vi "Energy Feedback Information Systems.vi"() -> ()   [LabVIEW 2014]
panel:
  in  "Path to Image":path=path "P:/My Documents/Demola/Naveen/Capture.PNG"
  out "t(s)":dbl
  in  "from 0s":bool
  in  "?":T1(tab)
  out "Suggested Actions":string
  out "Oil temperature meter":dbl(knob) scale=0.0..100.0
  out "Fuel meter":dbl(knob) scale=0.0..100.0
  out "Fuel Rate":dbl(slide) scale=0.0..75.0
  out "Bucket Fill (%)":dbl(knob) scale=0.0..100.0
  out "RPM Gauge":dbl(knob) scale=0.0..3000.0
  in  "Choose Excavator":string(combo)
  in  "Choose Cycles":u16(ring) items=["32", "16", "8", "4", "2", "1", ""]
  in  "Choose Driver":string(combo)
  out "Fuel Efficiency, [Kg/l]":cluster{dbl[], dbl[]}(graph)
  out "Torque/RPM Graph":cluster{dbl[], dbl[]}(graph)
  out "Time Productivity, [Kg/s]":cluster{dbl[], dbl[]}(graph)
  out "Dependence of best fuel consumption on engine RPM":i32[](graph)
  out "Dependencies of fuel consumption on filling % for 0 rpm Graph":i32[](graph)
  out "Dependence of best time productivity on engine RPM":i32[](graph)
  out "Dependencies of time productivity on filling % for 0 rpm":i32[](graph)
  out "Best Engine RPM":string
  out "Best filling %":string
  in  "Blank Button 2":bool
  in  "Blank Button":bool
  in  "Save Button 5":bool
  in  "Save Button 4":bool
  in  "Save Button 3":bool
  in  "Save Button 2":bool
  in  "Save Button":bool
  in  "String 6":string
  in  "String 5":string
  in  "String 4":string
  in  "String 3":string
  in  "Combo Box 5":string(combo)
  in  "Combo Box 4":string(combo)
  in  "Combo Box 3":string(combo)
  in  "Combo Box 2":string(combo)
  in  "Combo Box":string(combo)
  in  "String 2":string
  out "Check 1":dbl format="%#_10g"
  out "Check 4":dbl format="%#_10g"
  out "Check 2":dbl format="%#_10g"
  out "step":dbl
  out "Check 3":dbl format="%#_10g"
  out "millisecond timer value":u32
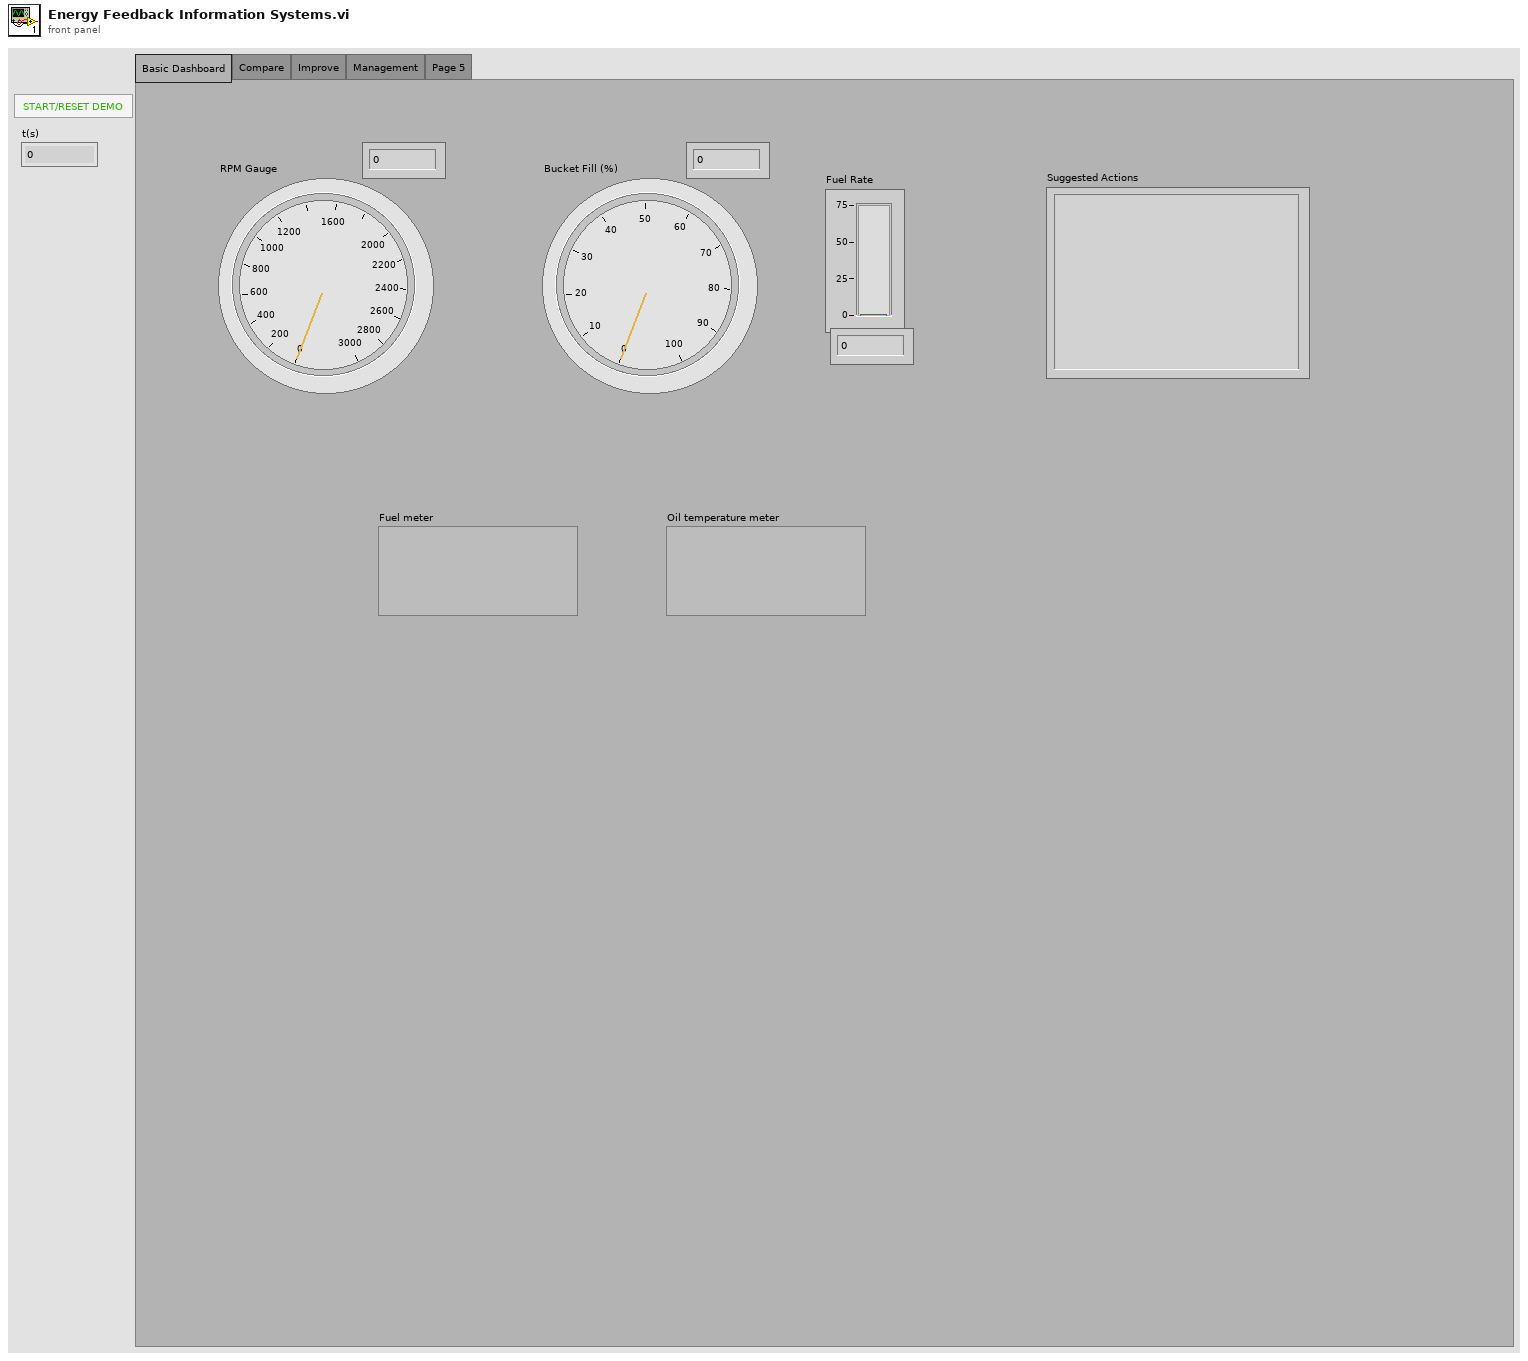
[diagram p1: front panel]
types:
  T1 = enum32{"Basic Dashboard", "Compare", "Improve", "Management", "Page 5"}
  T2 = typedef "imagedata.ctl" = cluster{"image type":i32, "image depth":i32, "image":u8[], "mask":u8[], "colors":u32[], "Rectangle":cluster{"left":i16, "top":i16, "right":i16, "bottom":i16}}
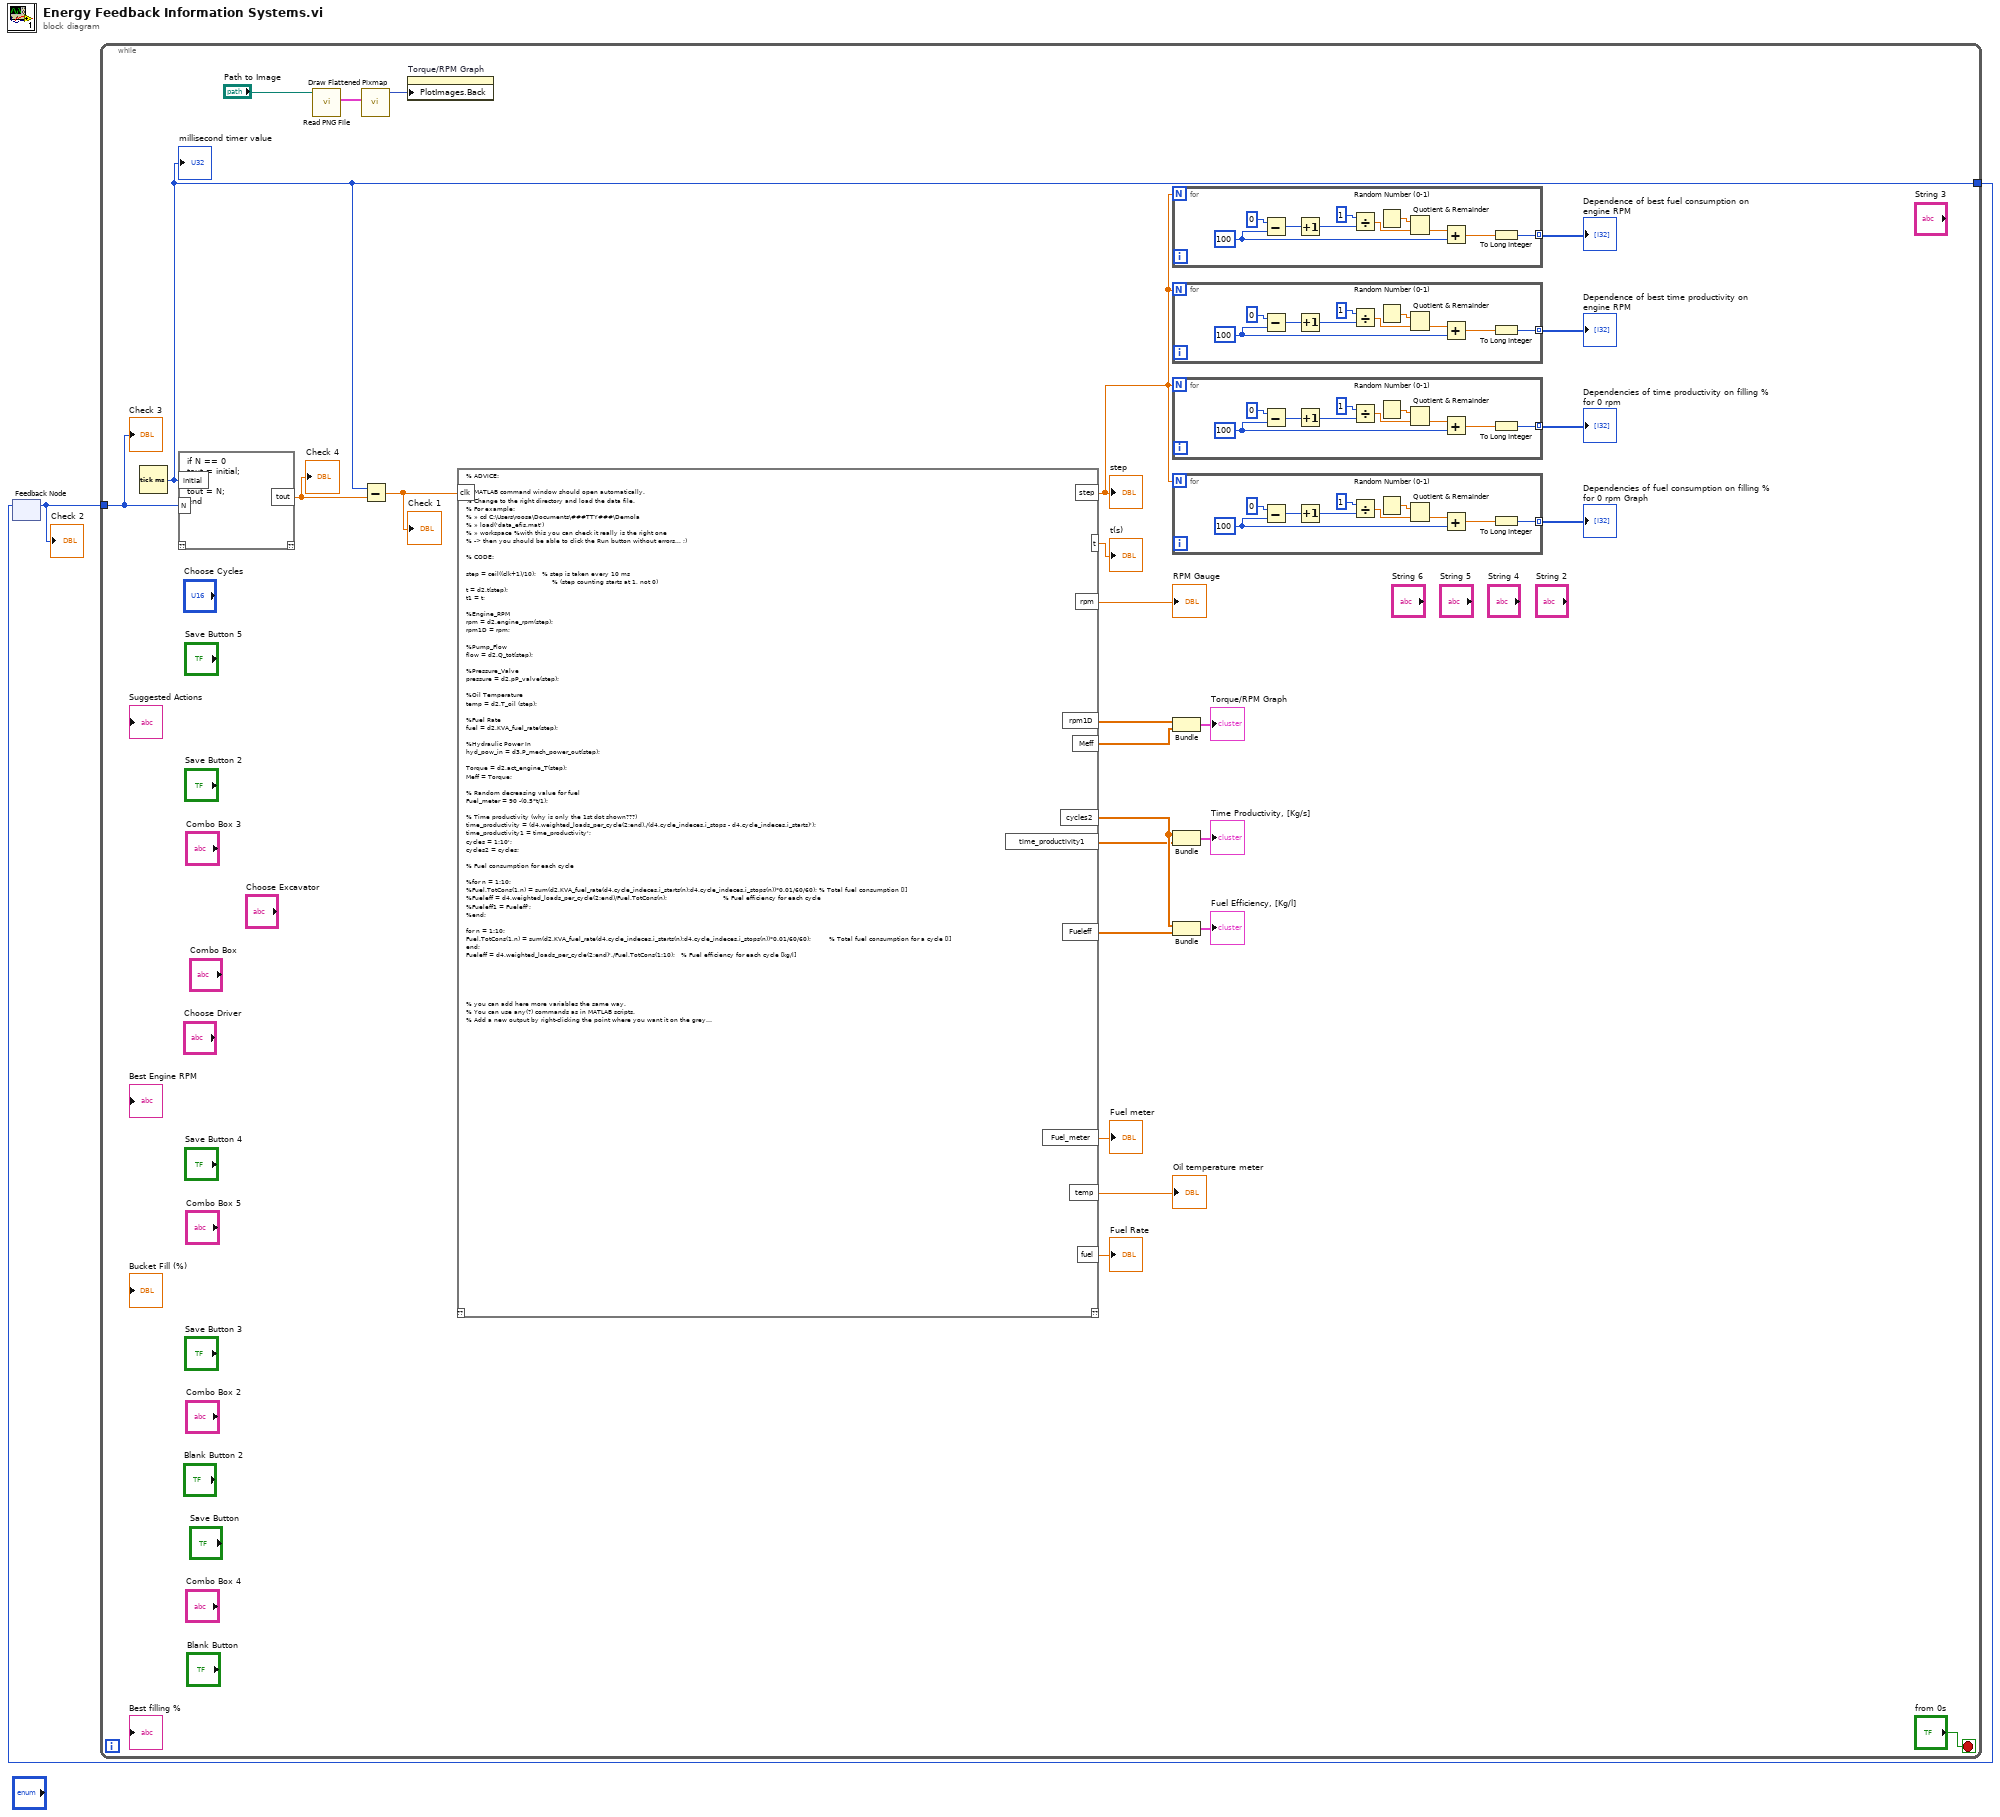
[diagram p0: block diagram]
diagram:
  n1 = feedback #1() -> (w1:u32)  [unwired: 1 in]
  "Check 2" <- w1
  n2 = while {
    tunnel: [w25] -> w2
    tunnel: w1 -> [w28]
    stop <- "from 0s" stop-if-true
    n3 = Tick Count (ms)() -> (millisecond timer value=w25:u32)
    "millisecond timer value" <- w25
    n4 = script code="if N == 0\ntout = initial;\nelse\ntout = N;\nend"("N"=w28, "initial"=w25) -> ("tout"=w27:dbl)  [unwired: 1 in, 1 out]
    "Check 4" <- w27
    n5 = call <vilib>:"Read PNG File.vi"("path to PNG file"="Path to Image") -> ("image data"=w12:T2)  [unwired: 8 in, 2 out]
    n6 = call <vilib>:"Draw Flattened Pixmap.vi"("image data"=w12) -> ("new picture"=w10:picture)  [unwired: 8 in]
    n7 = Subtract(x=w25, y=w27) -> (x-y=w26:dbl)
    "Check 1" <- w26
    n8 = property on="Torque/RPM Graph" class="XYGraph (strict)"("PlotImages.Back"=w10) -> ()  [unwired: 2 in, 2 out]
    n9 = script code="% ADVICE:\n\n% MATLAB command window should open automatically.\n% Change to the right directory and load the data file.\n% For example:\n% » cd C:\\Users\\roosa\\Documents\\###TTY###\\Demola\n% » load('data_efis.mat')\n% » workspace %with this you can check it really is the right one\n% -> then you should be able to click the Run button without errors... ;)\n\n% CODE:\n\nstep = ceil((clk+1)/10);   % step is taken every 10 ms \n                                           % (step counting starts at 1, not 0)\nt = d2.t(step);\nt1 = t;\n\n%Engine_RPM\nrpm = d2.engine_rpm(step);\nrpm1D = rpm;\n\n%Pump_Flow\nflow = d2.Q_tot(step);\n\n%Pressure_Valve\npressure = d2.pP_valve(step);\n\n%Oil Temperature\ntemp = d2.T_oil (step);\n\n%Fuel Rate\nfuel = d2.KVA_fuel_rate(step);\n\n%Hydraulic Power In\nhyd_pow_in = d3.P_mech_power_out(step);\n\nTorque = d2.act_engine_T(step);\nMeff = Torque;\n\n% Random decreasing value for fuel\nFuel_meter = 90 -(0.5*t/1);\n\n% Time productivity (why is only the 1st dot shown???)\ntime_productivity = (d4.weighted_loads_per_cycle(2:end)./(d4.cycle_indeces.i_stops - d4.cycle_indeces.i_starts)');\ntime_productivity1 = time_productivity';\ncycles = 1:10';\ncycles2 = cycles;\n\n% Fuel consumption for each cycle\n\n%for n = 1:10;\n%Fuel.TotCons(1,n) = sum(d2.KVA_fuel_rate(d4.cycle_indeces.i_starts(n):d4.cycle_indeces.i_stops(n))*0.01/60/60); % Total fuel consumption [l]\n%Fueleff = d4.weighted_loads_per_cycle(2:end)/Fuel.TotCons(n);                            % Fuel efficiency for each cycle\n%Fueleff1 = Fueleff';\n%end;\n\nfor n = 1:10;\nFuel.TotCons(1,n) = sum(d2.KVA_fuel_rate(d4.cycle_indeces.i_starts(n):d4.cycle_indeces.i_stops(n))*0.01/60/60);         % Total fuel consumption for a cycle [l]                          \nend;\t\t\nFueleff = d4.weighted_loads_per_cycle(2:end)'./Fuel.TotCons(1:10);   % Fuel efficiency for each cycle [kg/l]\n\n\n\n\n\n% you can add here more variables the same way.\n% You can use any(?) commands as in MATLAB scripts.\n% Add a new output by right-clicking the point where you want it on the grey bar there ->" ("Script Node")("clk"=w26) -> ("t"=→"t(s)":dbl, "step"=w4:dbl, "rpm"=→"RPM Gauge":dbl, "fuel"=→"Fuel Rate":dbl, "Meff"=w23:dbl[], "rpm1D"=w14:dbl[], "Fuel_meter"=→"Fuel meter":dbl, "temp"=→"Oil temperature meter":dbl, "time_productivity1"=w13:cdb[], "cycles2"=w16:dbl[], "Fueleff"=w17:dbl[])  [unwired: 1 in, 1 out]
    "step" <- w4
    n10 = for {
      N: w4 -> [_]
      tunnel: [w29] -> w5 mode=indexing
      w31 = 100
      n11 = Subtract(x=0, y=w31) -> (x-y=w38:i32)
      n12 = Increment(x=w38) -> (x+1=w37:i32)
      n13 = Divide(x=1, y=w37) -> (x/y=w32:dbl)
      n14 = Random Number (0-1)() -> (number: 0 to 1=w35:dbl)
      n15 = Quotient & Remainder(x=w35, y=w32) -> (floor(x/y)=w33:dbl)  [unwired: 1 out]
      n16 = Add(x=w33, y=w31) -> (x+y=w34:dbl)
      n17 = To Long Integer(number=w34) -> (32bit integer=w29:i32)
    }
    "Dependence of best fuel consumption on engine RPM" <- w5
    n18 = for {
      N: w4 -> [_]
      tunnel: [w49] -> w7 mode=indexing
      w51 = 100
      n19 = Subtract(x=0, y=w51) -> (x-y=w58:i32)
      n20 = Increment(x=w58) -> (x+1=w57:i32)
      n21 = Divide(x=1, y=w57) -> (x/y=w52:dbl)
      n22 = Random Number (0-1)() -> (number: 0 to 1=w55:dbl)
      n23 = Quotient & Remainder(x=w55, y=w52) -> (floor(x/y)=w53:dbl)  [unwired: 1 out]
      n24 = Add(x=w53, y=w51) -> (x+y=w54:dbl)
      n25 = To Long Integer(number=w54) -> (32bit integer=w49:i32)
    }
    "Dependence of best time productivity on engine RPM" <- w7
    n26 = for {
      N: w4 -> [_]
      tunnel: [w59] -> w9 mode=indexing
      w61 = 100
      n27 = Subtract(x=0, y=w61) -> (x-y=w68:i32)
      n28 = Increment(x=w68) -> (x+1=w67:i32)
      n29 = Divide(x=1, y=w67) -> (x/y=w62:dbl)
      n30 = Random Number (0-1)() -> (number: 0 to 1=w65:dbl)
      n31 = Quotient & Remainder(x=w65, y=w62) -> (floor(x/y)=w63:dbl)  [unwired: 1 out]
      n32 = Add(x=w63, y=w61) -> (x+y=w64:dbl)
      n33 = To Long Integer(number=w64) -> (32bit integer=w59:i32)
    }
    "Dependencies of time productivity on filling % for 0 rpm" <- w9
    n34 = for {
      N: w4 -> [_]
      tunnel: [w39] -> w6 mode=indexing
      w41 = 100
      n35 = Subtract(x=0, y=w41) -> (x-y=w48:i32)
      n36 = Increment(x=w48) -> (x+1=w47:i32)
      n37 = Divide(x=1, y=w47) -> (x/y=w42:dbl)
      n38 = Random Number (0-1)() -> (number: 0 to 1=w45:dbl)
      n39 = Quotient & Remainder(x=w45, y=w42) -> (floor(x/y)=w43:dbl)  [unwired: 1 out]
      n40 = Add(x=w43, y=w41) -> (x+y=w44:dbl)
      n41 = To Long Integer(number=w44) -> (32bit integer=w39:i32)
    }
    "Dependencies of fuel consumption on filling % for 0 rpm Graph" <- w6
    n42 = Bundle(w14, w23) -> (→"Torque/RPM Graph":cluster{dbl[], dbl[]})  [unwired: 1 in]
    n43 = Bundle(w16, w13) -> (→"Time Productivity, [Kg/s]":cluster{dbl[], cdb[]})  [unwired: 1 in]
    n44 = Bundle(w16, w17) -> (→"Fuel Efficiency, [Kg/l]":cluster{dbl[], dbl[]})  [unwired: 1 in]
    "Check 3" <- w28
  }
  n45 = feedback-in #1(w2) -> ()
